vi "TempRefnum.vi"(1 "change?":bool, 2 "refnum in":refnum<k1>) -> (0 "refnum out":refnum<k1>)   [LabVIEW 2009]
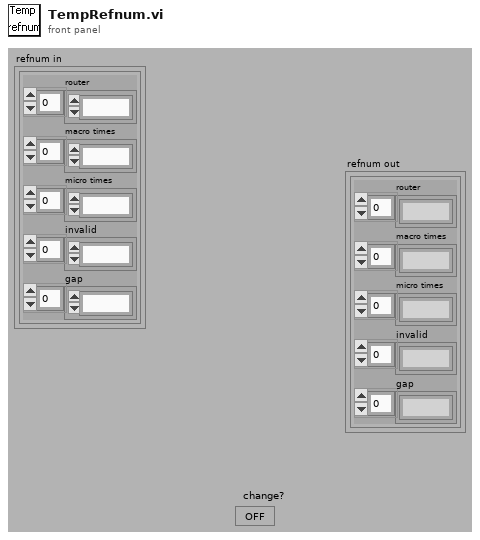
[diagram p1: front panel]
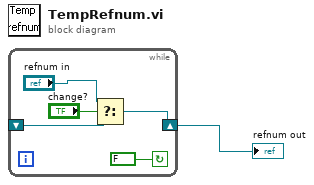
[diagram p0: block diagram]
diagram:
  n1 = while {
    shift-right: [w5] -> w1
    shift-left: _ -> [w6]
    stop <- FALSE continue-if-true
    n2 = Select(t="refnum in", s="change?", f=w6) -> (s? t:f=w5:refnum<k1>)
  }
  "refnum out" <- w1
